vi "getZTAACTestSetting.vi"() -> (3 "Test Setting":T2)   [LabVIEW 2016]
doc: "Get the test setting of ZTAAC class."
uses:
  StrictDef/InstName.ctl
  OfcFunc.lvlib
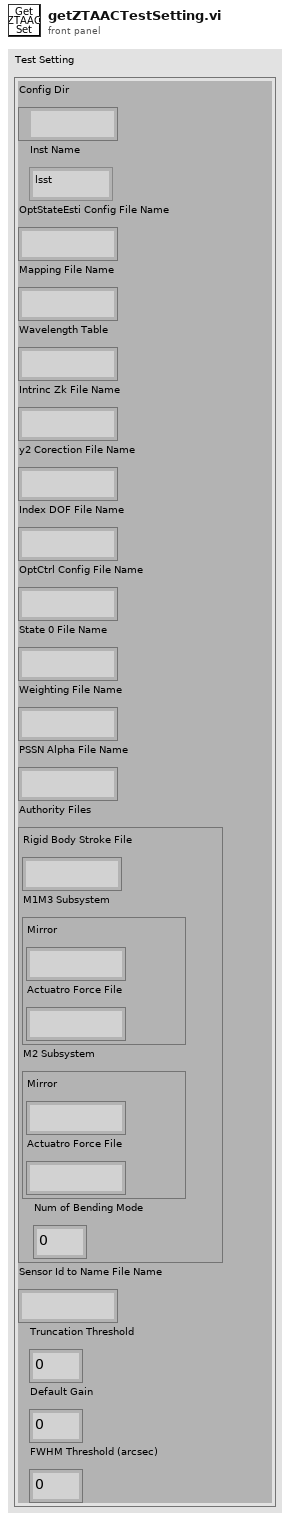
[diagram p1: front panel]
types:
  T1 = typedef "OfcFunc.lvlib/InstName.ctl" = enum16{"lsst", "comcam"}
  T2 = cluster{"Config Dir":path, "Inst Name":T1, "OptStateEsti Config File Name":string, "Mapping File Name":string, "Wavelength Table":string, "Intrinc Zk File Name":string, "y2 Corection File Name":string, "Index DOF File Name":string, "OptCtrl Config File Name":string, "State 0 File Name":string, "Weighting File Name":string, "PSSN Alpha File Name":string, "Authority Files":cluster{"Rigid Body Stroke File":string, "M1M3 Subsystem":cluster{"Mirror":string, "Actuatro Force File":string}, "M2 Subsystem":cluster{"Mirror":string, "Actuatro Force File":string}, "Num of Bending Mode":i32}, "Sensor Id to Name File Name":string, "Truncation Threshold":dbl, "Default Gain":dbl, "FWHM Threshold (arcsec)":dbl}
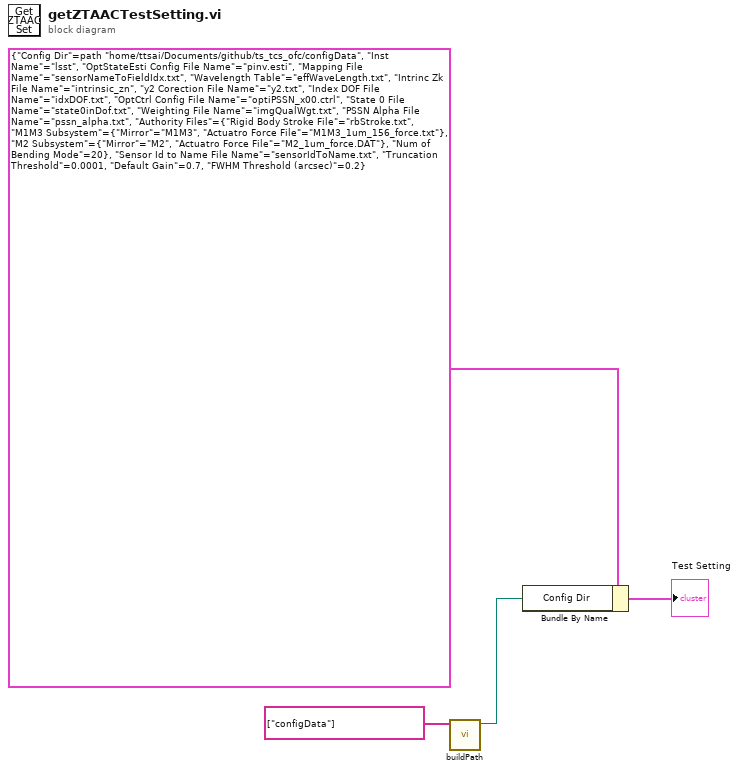
[diagram p0: block diagram]
diagram:
  n1 = call "buildPath.vi"("Path Name List"=string[] ["configData"]) -> ("New Path"=w3:path)  [unwired: 10 in]
  n2 = Bundle By Name(cluster=T2 {"Config Dir"=path "/home/ttsai/Documents/github/ts_tcs_ofc/configData", "Inst Name"=enum."lsst", "OptStateEsti Config File Name"="pinv.esti", "Mapping File Name"="sensorNameToFieldIdx.txt", "Wavelength Table"="effWaveLength.txt", "Intrinc Zk File Name"="intrinsic_zn", "y2 Corection File Name"="y2.txt", "Index DOF File Name"="idxDOF.txt", "OptCtrl Config File Name"="optiPSSN_x00.ctrl", "State 0 File Name"="state0inDof.txt", "Weighting File Name"="imgQualWgt.txt", "PSSN Alpha File Name"="pssn_alpha.txt", "Authority Files"={"Rigid Body Stroke File"="rbStroke.txt", "M1M3 Subsystem"={"Mirror"="M1M3", "Actuatro Force File"="M1M3_1um_156_force.txt"}, "M2 Subsystem"={"Mirror"="M2", "Actuatro Force File"="M2_1um_force.DAT"}, "Num of Bending Mode"=20}, "Sensor Id to Name File Name"="sensorIdToName.txt", "Truncation Threshold"=0.0001, "Default Gain"=0.7, "FWHM Threshold (arcsec)"=0.2} ("ZTAAC Configuration"), "Config Dir"=w3) -> (→"Test Setting":T2)
